vi "1-3.1 클릭반응시간_UserInterfaceEventPattern 4.vi"() -> ()   [LabVIEW 2014]
doc: "이 템플릿을 사용하여 사용자 인터페이스 이벤트 핸들러 디자인 패턴을 생성합니다. 대화 상자 및 다른 사용자 인터페이스에 대하여 이 패턴을 사용합니다. 또한, VI가 사용자 인터페이스 이벤트를 같은 방법으로 다룰 수 있는, 사용자 정의 이벤트를 생성하고 실행할 수 있습니다."
panel:
  out "시간측정":dbl
  in  "확인 버튼":bool
  in  "정지":bool
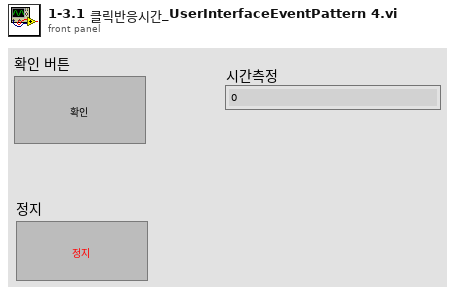
[diagram p1: front panel]
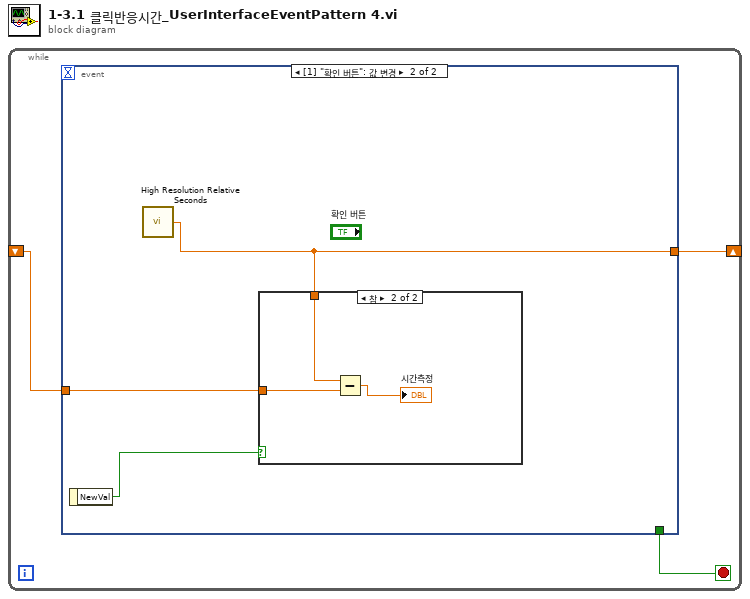
[diagram p0: block diagram]
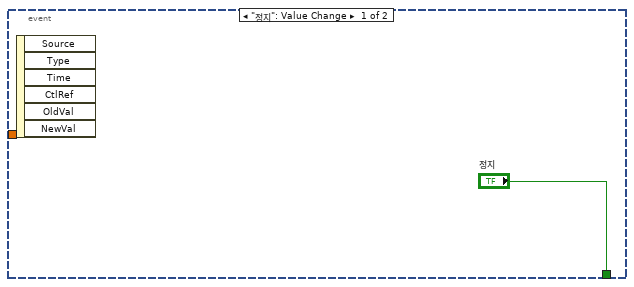
[diagram p2: hidden frame]
diagram:
  n1 = while {
    shift-right: [w2] -> _
    shift-left: _ -> [w1]
    stop <- w3 stop-if-true
    n2 = event shown="[1] \"확인 버튼\": 값 변경" {
      selector: _ -> [_ _]
      dyn-events: _ -> [_ _]
      timeout: _ -> [_ _]
      tunnel: ["정지" _] -> w3
      tunnel: [_ w5] -> w2
      tunnel: w1 -> [_ w6]
      event "정지": Value Change {
        n3 = event-data() -> ()  [unwired: 1 in, 6 out]
      }
      event "확인 버튼": Value Change {
        n4 = event-data() -> ("NewVal"=w7:bool)  [unwired: 1 in]
        n5 = call <vilib>:"High Resolution Relative Seconds.vi"() -> ("relative seconds"=w5:dbl)
        n6 = case shown="참" w7 {
          tunnel: w5 -> [_ w10]
          tunnel: w6 -> [_ w8]
          frame False {
          }
          frame True {
            n7 = Subtract(x=w10, y=w8) -> (x-y=→"시간측정":dbl)
          }
        }
      }
    }
  }
